vi "DS_Calc_and_Normalize_by_Self_Stats.vi"(11 "DS in":sgl[][][][](array[numeric])) -> (3 "DS out":sgl[][][][](array[numeric]), 5 "Dataset_Stats":T1={"means"={"R"=0.5401046, "G"=0.5370146, "B"=0.5527349}, "stds"={"R"=0.36788714, "G"=0.36817855, "B"=0.35177523}} {"stds"."R" format="%#_3g"; "stds"."G" format="%#_3g"; "stds"."B" format="%#_3g"; "means"."R" format="%#_3g"; "means"."G" format="%#_3g"; "means"."B" format="%#_3g"})   [LabVIEW 2024]
uses:
  <vilib>/Ngene/DeepLTK Anomaly Detection Addon/DeepLTK_Anomaly_Detection_Addon/API/Controls/NNPC_DS_Stats.ctl
  <vilib>/Ngene/DeepLTK Anomaly Detection Addon/DeepLTK_Anomaly_Detection_Addon/API/Controls/Image_Stats_RGB.ctl
  <vilib>/Ngene/DeepLTK Anomaly Detection Addon/DeepLTK_Anomaly_Detection_Addon/DeepLTK_Anomaly_Detection_Addon.lvlib
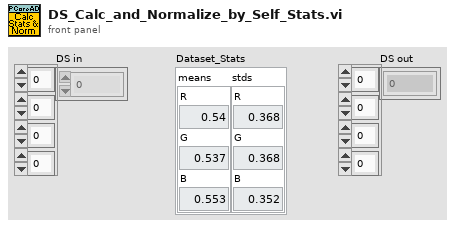
[diagram p1: front panel]
types:
  T1 = typedef "DeepLTK_Anomaly_Detection_Addon.lvlib/NNPC_DS_Stats.ctl" = cluster{"means":T2, "stds":T2}
  T2 = typedef "DeepLTK_Anomaly_Detection_Addon.lvlib/Image_Stats_RGB.ctl" = cluster{"R":sgl, "G":sgl, "B":sgl}
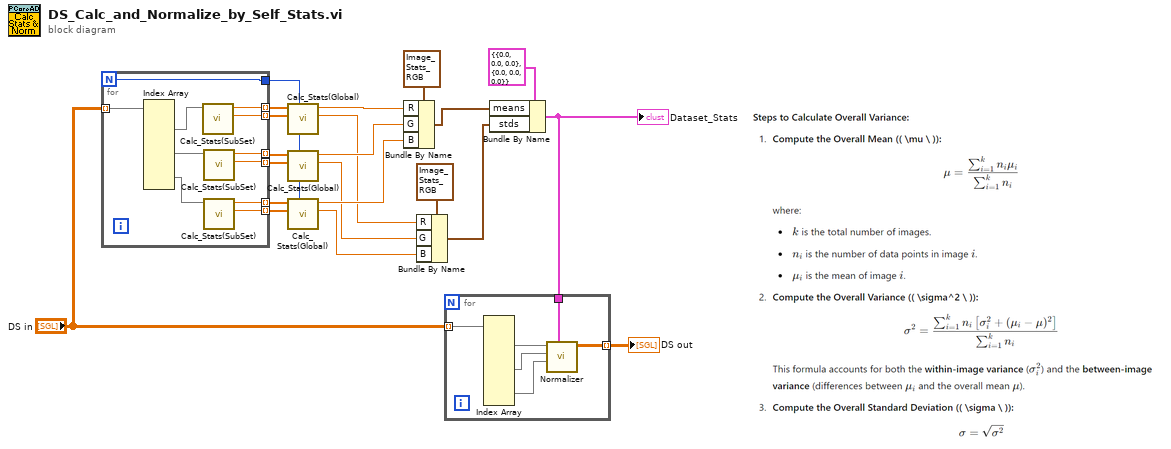
[diagram p0: block diagram]
diagram:
  n1 = for {
    N -> [w32]
    tunnel: [w32] -> w10
    tunnel: [w28] -> w12 mode=indexing
    tunnel: [w27] -> w9 mode=indexing
    tunnel: [w26] -> w7 mode=indexing
    tunnel: [w25] -> w11 mode=indexing
    tunnel: [w23] -> w8 mode=indexing
    tunnel: [w24] -> w6 mode=indexing
    tunnel: "DS in" -> [w22] mode=indexing
    n2 = Index Array(array=w22) -> (element #1=w31:sgl[][], element #2=w30:sgl[][], element #3=w29:sgl[][])  [unwired: 9 in]
    n3 = call "Calc_Stats(SubSet).vi"("Image Out"=w31) -> ("variance"=w25:sgl, "mean"=w28:sgl)  [unwired: 8 in, 1 out]
    n4 = call "Calc_Stats(SubSet).vi"("Image Out"=w30) -> ("variance"=w23:sgl, "mean"=w27:sgl)  [unwired: 8 in, 1 out]
    n5 = call "Calc_Stats(SubSet).vi"("Image Out"=w29) -> ("variance"=w24:sgl, "mean"=w26:sgl)  [unwired: 8 in, 1 out]
  }
  n6 = call "Calc_Stats(Global).vi"("No of SubSets"=w10, "Local Vars"=w11, "Local Means"=w12) -> ("Global STD"=w3:sgl, "Global Mean"=w18:sgl)  [unwired: 7 in]
  n7 = call "Calc_Stats(Global).vi"("No of SubSets"=w10, "Local Vars"=w8, "Local Means"=w9) -> ("Global STD"=w2:sgl, "Global Mean"=w5:sgl)  [unwired: 7 in]
  n8 = call "Calc_Stats(Global).vi"("No of SubSets"=w10, "Local Vars"=w6, "Local Means"=w7) -> ("Global STD"=w1:sgl, "Global Mean"=w4:sgl)  [unwired: 7 in]
  n9 = Bundle By Name(cluster=T2 {"R"=0.66, "G"=0.59, "B"=0.44} ("means"), "R"=w18, "G"=w5, "B"=w4) -> (w16:T2)
  n10 = Bundle By Name(cluster=T2 {"R"=0.66, "G"=0.59, "B"=0.44} ("means"), "R"=w3, "G"=w2, "B"=w1) -> (w15:T2)
  n11 = Bundle By Name(cluster=T1 {"means"={"R"=0.0, "G"=0.0, "B"=0.0}, "stds"={"R"=0.0, "G"=0.0, "B"=0.0}} ("Dataset_Stats"), "means"=w16, "stds"=w15) -> (w14:T1)
  "Dataset_Stats" <- w14
  n12 = for {
    tunnel: "DS in" -> [w38] mode=indexing
    tunnel: w14 -> [w34]
    tunnel: [w33] -> w13 mode=indexing
    n13 = Index Array(array=w38) -> (element #1=w37:sgl[][], element #2=w36:sgl[][], element #3=w35:sgl[][])  [unwired: 9 in]
    n14 = call "Normalizer.vi"("Dataset_Stats"=w34, "B"=w35, "G"=w36, "R"=w37) -> ("Norm_Img_Out"=w33:sgl[][][])  [unwired: 7 in]
  }
  "DS out" <- w13
